vi "State_Machine.vi"(8 "error in (no error)":errorcluster caption="entrée d'erreur (pas d'erreur)", 11 "Get_Voltage en entrée":refnum<class "Zigbee_Network_Creator.lvclass">) -> (0 "error out":errorcluster caption="sortie d'erreur", 2 "Json_String":string, 3 "Get_Voltage en sortie":refnum<class "Zigbee_Network_Creator.lvclass">)   [LabVIEW 2020, in "Library Test.lvlib" / "Zigbee_Network_Creator.lvclass"]
uses:
  Zigbee_Network_Creator.lvclass
  C:/Users/ngarcin/OneDrive - Altyor/Standard TB/Class/Test/Test (Default)/Test (Default).lvclass
  C:/Users/ngarcin/OneDrive - Altyor/Standard TB/Class/Test/Zigbee_Send_Command_UART/Zigbee_Send_Command_UART.lvclass
  <vilib>/numeric/Random Number (Range) U64.vi
  <vilib>/numeric/sub_Random U32.vi
  Zigbee_Send_Command_UART/Zigbee_Send_Command_UART.lvclass
  Zigbee_Network_Creator.lvclass/Zigbee_Network_Creator.ctl
  Commun VI/Library Commun.lvlib
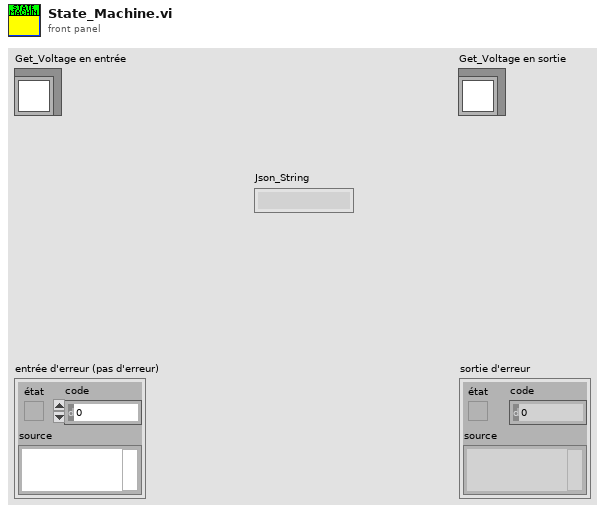
[diagram p1: front panel]
types:
  T1 = enum16{"CRC Altyor", "CRC Xor On all Bytes", "CRC8", "CRC16", "CRC32", "Other"}
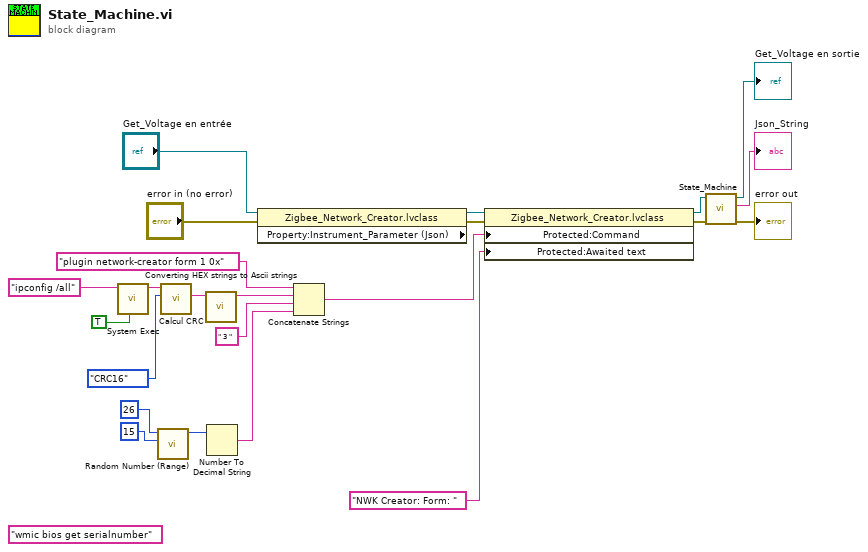
[diagram p0: block diagram]
diagram:
  (unwired) "wmic bios get serialnumber" ("command line")
  n1 = call <vilib>:"System Exec.vi"("run minimized? (F)"=TRUE, "command line"="ipconfig /all") -> ("standard output"=w11:string)  [unwired: 6 in, 3 out]
  n2 = call-poly <vilib>:"Random Number (Range).vi"("lower bound (0)"=u64 15, "upper bound (100)"=u64 26) -> ("number"=w14:u64)  [unwired: 9 in]
  n3 = call "Calcul CRC.vi"("CRC type"=T1."CRC16", "Trame"=w11) -> ("CRC"=w2:string)  [unwired: 8 in, 1 out]
  n4 = call "Converting HEX strings to Ascii strings.vi"("chaîne IN"=w2) -> ("Chaîne OUT"=w1:string)  [unwired: 9 in, 1 out]
  n5 = Number To Decimal String(number=w14) -> (decimal integer string=w13:string)  [unwired: 1 in]
  n6 = property class="Zigbee_Network_Creator.lvclass" props=["Property:Instrument_Parameter (Json)"](reference="Get_Voltage en entrée", error in="error in (no error)") -> (reference out=w20:refnum<class "Zigbee_Network_Creator.lvclass">, error out=w8:errorcluster)  [unwired: 1 out]
  n7 = Concatenate Strings("plugin network-creator form 1 0x" ("Command"), w1, " 3 " ("chaîne"), w13) -> (w17:string)
  n8 = property class="Zigbee_Network_Creator.lvclass"(reference=w20, error in=w8, "Protected:Command"=w17, "Protected:Awaited text"="NWK Creator: Form: " ("Awaited text")) -> (reference out=w4:refnum<class "Zigbee_Network_Creator.lvclass">, error out=w5:errorcluster)
  n9 = call-parent "State_Machine.vi"("error in (no error)"=w5, "Send_Frame en entrée"=w4) -> ("error out"=→"error out":errorcluster, "Json_String"=→"Json_String":string, "Send_Frame en sortie"=→"Get_Voltage en sortie":refnum<class "Zigbee_Network_Creator.lvclass">)  [unwired: 7 in]
